vi "Main.vi"() -> ()   [LabVIEW 2017]
doc: "The myRIO Project template acquires acceleration data from the onboard accelerometer and displays the changes of acceleration values in a waveform chart."
uses:
  <vilib>/myRIO/Instrument Drivers/Onboard IO/DIO/typedefs/DIO Reference.ctl
  <vilib>/myRIO/Common/Instrument Driver Framework/Utilities/typedefs/myRIO Generic Hardware Reference.ctl
  <vilib>/myRIO/Common/Instrument Driver Framework/Utilities/typedefs/Hardware Version Enum.ctl
  <vilib>/myRIO/Common/Instrument Driver Framework/Utilities/typedefs/myRIO v1.0 Reference.ctl
  <vilib>/myRIO/Common/Instrument Driver Framework/Utilities/typedefs/Generic FPGA Reference.ctl
  <vilib>/myRIO/Common/Instrument Driver Framework/myRIO v1.0/DIO/typedefs/DIO Channels List.ctl
  <vilib>/myRIO/Common/Instrument Driver Framework/myRIO v1.0/DIO/typedefs/DIO Channels Enum.ctl
  <vilib>/userdefined/High Color/nirio_resource_hc.ctl
  <vilib>/myRIO/Instrument Drivers/Onboard IO/UART/typedef/VISA Configuration.ctl
  <vilib>/myRIO/Common/Instrument Driver Framework/Utilities/vis/Is FPGA Ref Available.vi
  <vilib>/myRIO/Common/Instrument Driver Framework/myRIO v1.0/DIO/vis/myRIO v1.1 Open DIO.vi
  <vilib>/myRIO/Instrument Drivers/Onboard IO/DIO/vis/Write.vi
  <vilib>/myRIO/Instrument Drivers/Onboard IO/DIO/vis/Read.vi
  <vilib>/myRIO/Common/Instrument Driver Framework/Utilities/vis/Validate Channels.vi
  <vilib>/myRIO/Common/Instrument Driver Framework/myRIO v1.0/DIO/vis/myRIO v1.0 Reserve DIO.vi
  <vilib>/myRIO/Common/Instrument Driver Framework/myRIO v1.0/UART/vis/myRIO v1.0 Close UART.vi
  <vilib>/myRIO/Common/Instrument Driver Framework/myRIO v1.0/Resource Manager/vis/myRIO v1.0 Reserve Channel List.vi
  <vilib>/myRIO/Common/Instrument Driver Framework/myRIO v1.0/DIO/vis/myRIO v1.0 Build MUX Configuration DIO.vi
  <vilib>/myRIO/Common/Instrument Driver Framework/myRIO v1.0/Resource Manager/vis/myRIO v1.0 Reserve Channel.vi
  <vilib>/myRIO/Common/Instrument Driver Framework/myRIO v1.0/Resource Manager/vis/myRIO v1.0 Unreserve Channel.vi
  <vilib>/myRIO/Common/Instrument Driver Framework/myRIO v1.0/Resource Manager/vis/myRIO v1.0 Create Configuration List.vi
  <vilib>/myRIO/Common/Instrument Driver Framework/myRIO v1.0/Resource Manager/vis/myRIO v1.0 Build Mutex Name.vi
  <vilib>/Utility/VariantDataType/GetNumericInfo.vi
  <vilib>/Utility/error.llb/Error Cluster From Error Code.vi
  <vilib>/myRIO/Common/Instrument Driver Framework/myRIO v1.0/myRIO v1.1 Open.vi
  <vilib>/myRIO/Common/Instrument Driver Framework/Utilities/vis/IO Manager.vi
  <vilib>/myRIO/Common/Instrument Driver Framework/Utilities/vis/Configuration Manager.vi
  <vilib>/myRIO/Common/Instrument Driver Framework/myRIO v1.0/Resource Manager/vis/myRIO v1.0 Configure IO.vi
  <vilib>/myRIO/Common/Instrument Driver Framework/myRIO v1.0/myRIO v1.0 Close.vi
  <vilib>/myRIO/Common/Instrument Driver Framework/myRIO v1.0/DIO/vis/myRIO v1.0 Write DIO.vi
  <vilib>/Instr/_visa.llb/VISA Configure Serial Port (Instr).vi
  <vilib>/myRIO/Common/Instrument Driver Framework/myRIO v1.0/DIO/vis/myRIO v1.0 Read DIO.vi
  <vilib>/Utility/file.llb/Write Delimited Spreadsheet (string).vi
  <vilib>/myRIO/Common/Instrument Driver Framework/Utilities/vis/FPGA Ref Manager.vi
  <vilib>/myRIO/Common/Instrument Driver Framework/myRIO v1.0/myRIO v1.0 Reset FPGA.vi
  <vilib>/myRIO/Common/Instrument Driver Framework/myRIO v1.0/IRQ/vis/myRIO v1.0 IRQ Info FGV.vi
  <vilib>/myRIO/Common/Instrument Driver Framework/myRIO v1.0/IRQ/vis/myRIO v1.0 Timer IRQ Info FGV.vi
  <vilib>/myRIO/Common/Instrument Driver Framework/myRIO v1.0/IRQ/vis/myRIO v1.0 ISR Agent.vi
  <vilib>/myRIO/Express VI/Onboard IO/DO/DO Express VI.xnode
  <vilib>/myRIO/Instrument Drivers/Onboard IO/DIO/vis/myRIO DIO Open.xnode
  <vilib>/myRIO/Express VI/Onboard Devices/LED/LED Express VI.xnode
  <vilib>/myRIO/Express VI/Onboard IO/UART/UART Express VI.xnode
  <vilib>/myRIO/Express VI/Onboard IO/DI/DI Express VI.xnode
  <vilib>/myRIO/Express VI/Onboard Devices/Button/Button Express VI.xnode
  <vilib>/myRIO/Instrument Drivers/Utilities/Utilities.lvlib
  <vilib>/myRIO/Instrument Drivers/Onboard IO/UART/UART.lvlib
  <vilib>/myRIO/Instrument Drivers/Onboard IO/DIO/DIO.lvlib
panel:
  out "LinkIt Response\nTimed Out 3":bool
  out "time to \nrespond":dbl
  out "DIO Failure":bool
  out "System Log":string
  out "Data Log":string[](array[string])
  out "System Log Write Path":path
  out "Data Log Write Path":path
  out "Pin 11 State":bool
  out "Pin 13 State":bool
  out "Message Received":string
  out "Message to Send":string
  out "Time to Send \nMessage":dbl
  out "LinkIt Response\nTimed Out 2":bool
  out "LinkIt Response\nTimed Out 1":bool
  out "Data Queue Error":bool
  out "LinkIt Failure":bool
  out "Initialisation \nsuccessfull":bool
  out "Storage Device Failure":bool
  out "D.L.B. Status":bool
  out "?":i32(slide) scale=0.1..100.0
  out "?":bool
  out "?":bool
  out "?":bool
  out "?":bool
  out "S.L.H. Status":bool
  out "S.L.B. Status":bool
  out "S.L. Status":bool
  out "D.L.H. Status":bool
  out "M.S. Status":bool
  out "M.H. Status":bool
  out "M.R. Status":bool
  out "System Uptime":string
  in  "Array":string[](array[string])
  out "error out":errorcluster
  in  "Stop":bool
  # "Overview: The myRIO Project template acquires acceleration data from the onboard accelerometer and displays the changes of acceleration values in a waveform chart.\nInstructions:\n1. Check the myRIO target IP address in the project and make sure the target IP address is correct. \n2. Run this VI."
  # "Signal Level"
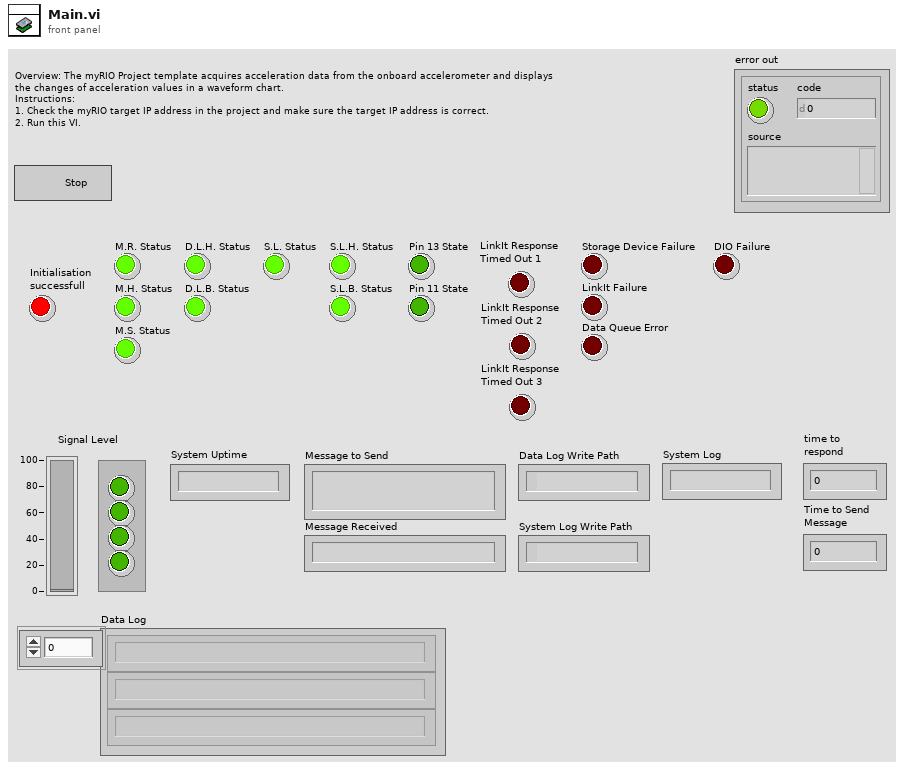
[diagram p1: front panel]
types:
  T1 = cluster{string, string, string, string, string, string, string, string, string, string}
  T2 = typedef "DIO.lvlib/DIO Reference.ctl" = cluster{"myRIO Reference":T3, "DIO Channels List":T7}
  T3 = typedef "myRIO Generic Hardware Reference.ctl" = cluster{"myRIO Model":T4, "myRIO Hardware Reference":T5}
  T4 = typedef "Hardware Version Enum.ctl" = enum16{"Unknown", "myRIO-1900", "myRIO-1950", "roboRIO", "NI ELVIS RIO CM"}
  T5 = typedef "myRIO v1.0 Reference.ctl" = cluster{"Generic FPGA Reference":T6, "Allow multiple opens":bool}
  T6 = typedef "Generic FPGA Reference.ctl" = refnum<k20>
  T7 = typedef "DIO Channels List.ctl" = T8[]
  T8 = typedef "DIO Channels Enum.ctl" = enum16{"Not Connected", "C/DIO0", "C/DIO1", "C/DIO2", "C/DIO3", "C/DIO4", "C/DIO5", "C/DIO6", "C/DIO7", "A/DIO0", "A/DIO1", "A/DIO2", "A/DIO3", "A/DIO4", "A/DIO5", "A/DIO6", "A/DIO7", "A/DIO8", "A/DIO9", "A/DIO10", "A/DIO11", "A/DIO12", "A/DIO13", "A/DIO14", "A/DIO15", "B/DIO0", "B/DIO1", "B/DIO2", "B/DIO3", "B/DIO4", "B/DIO5", "B/DIO6", "B/DIO7", "B/DIO8", "B/DIO9", "B/DIO10", "B/DIO11", "B/DIO12", "B/DIO13", "B/DIO14", "B/DIO15", "LED0", "LED1", "LED2", "LED3", "Button0", "DIO/DIO0", "DIO/DIO1", "DIO/DIO2", "DIO/DIO3", "DIO/DIO4", "DIO/DIO5", "DIO/DIO6", "DIO/DIO7", "DIO/DIO8", "DIO/DIO9", "SPI/CS0", "SPI/CS1", "SPI/CS2", "SPI/CS3", "LED RADIO (Green)", "LED RADIO (Red)", "LED COMM (Green)", "LED COMM (Red)", "LED MODE (Green)", "LED MODE (Red)"}
  T9 = typedef "nirio_resource_hc.ctl" = tag
  T10 = typedef "UART.lvlib/VISA Configuration.ctl" = cluster{"baud rate (9600)":u32, "data bits (8)":u16, "parity (0:none)":enum16{"None", "Odd", "Even", "Mark", "Space"}, "stop bits (10: 1 bit)":u16, "flow control (0:none)":u16, "termination char\n(0xA = '\\n' = LF) ":u8, "Enable Termination\nChar (T)":bool, "timeout (10sec)":u32}
  T11 = enum16{"open", "replace", "create", "open or create", "replace or create", "replace or create with confirmation"}
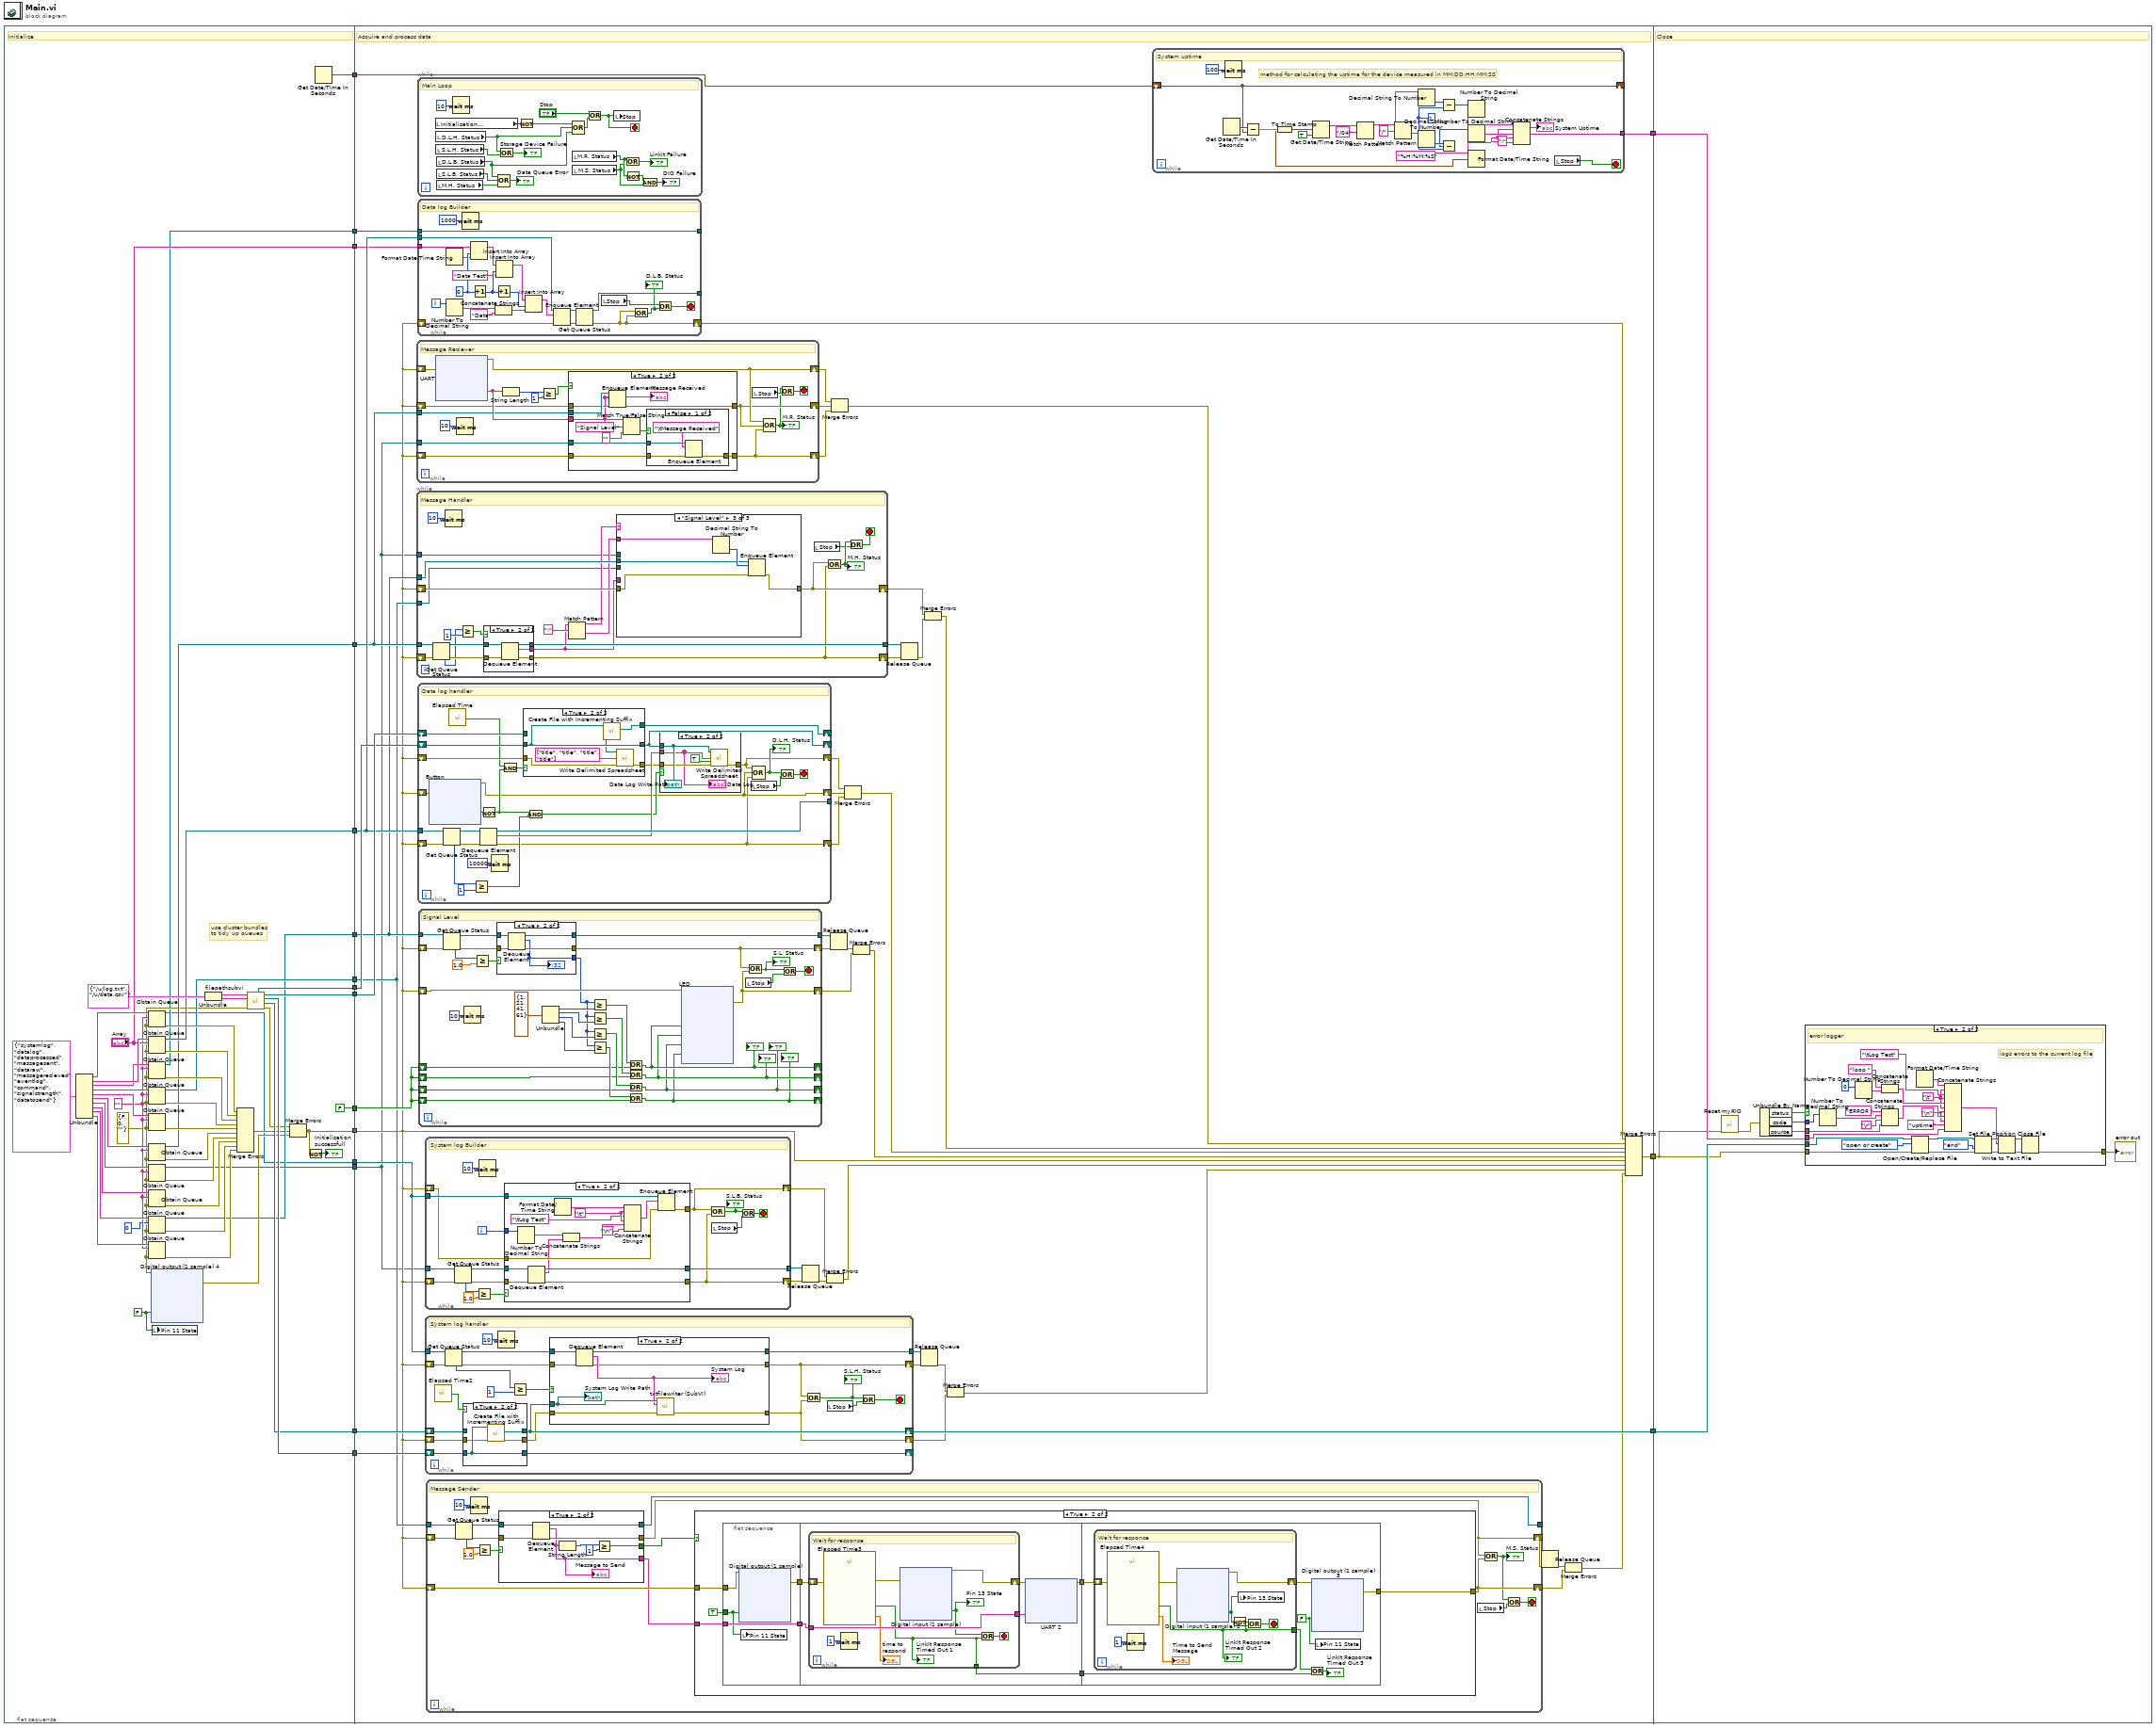
[diagram p0: block diagram]
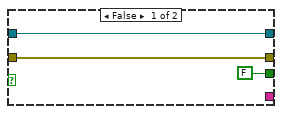
[diagram p3: hidden frame]
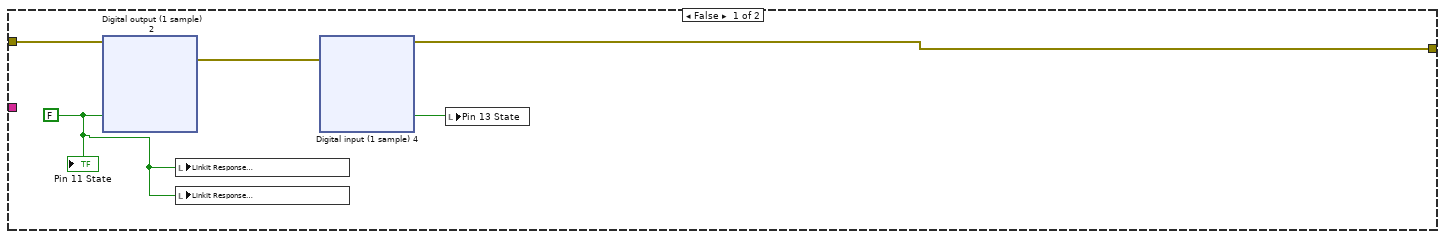
[diagram p4: hidden frame]
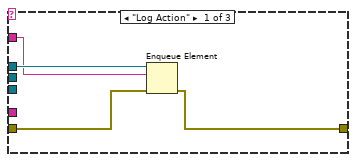
[diagram p6: hidden frame]
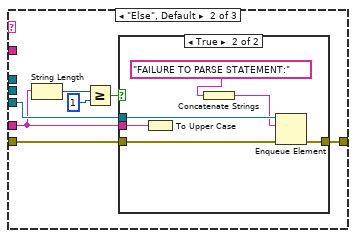
[diagram p7: hidden frame]
diagram:
  n1 = flat-sequence {
    tunnel: [w64] -> w17
    tunnel: [w55] -> w16
    tunnel: [w21] -> w15
    tunnel: [w54] -> w14
    tunnel: [w53] -> w13
    tunnel: [w19] -> w12
    tunnel: ["Array"] -> w11
    tunnel: [w20] -> w10
    tunnel: [w37] -> w9
    tunnel: [w36] -> w8
    tunnel: [w34] -> w6
    tunnel: [w33] -> w5
    tunnel: [w31] -> w4
    tunnel: [w30] -> w3
    tunnel: [FALSE] -> w2
    tunnel: [w152] -> w18
    tunnel: w17 -> [w151]
    tunnel: w16 -> [w148]
    tunnel: w15 -> [w111]
    tunnel: w14 -> [w150]
    tunnel: w13 -> [w149]
    tunnel: w12 -> [w141]
    tunnel: w11 -> [w147]
    tunnel: w10 -> [w146]
    tunnel: w9 -> [w145]
    tunnel: w8 -> [w144]
    tunnel: [w143] -> w7
    tunnel: w6 -> [w142]
    tunnel: w5 -> [w113]
    tunnel: w4 -> [w102]
    tunnel: w3 -> [w116]
    tunnel: w2 -> [w138]
    tunnel: [w101] -> w1
    tunnel: w18 -> [w857]
    tunnel: w7 -> [w854]
    tunnel: w1 -> [w853]
    frame #0 {
      w24 = FALSE
      w32 = ""
      w23 = errorcluster {"status"=FALSE, "code"=0, "source"=""} ("error in (no error)")
      # "use cluster bundles\nto tidy up queues"
      # "Initialize"
      n2 = Unbundle(T1 {"systemlog", "datalog", "dataprocessed", "messagesent", "dataraw", "messagerecieved", "eventlog", "command", "signalstrength", "datatosend"}) -> (w60:string, w59:string, w58:string, w57:string, w56:string, w47:string, w45:string, w44:string, w43:string, w42:string)
      n3 = Obtain Queue(name (unnamed)=w60, element data type=w32, error in (no error)=w23) -> (queue out=w19:refnum<queue>, error out=w52:errorcluster)  [unwired: 2 in, 1 out]
      n4 = Obtain Queue(name (unnamed)=w59, element data type="Array", error in (no error)=w23) -> (queue out=w55:refnum<queue>, error out=w51:errorcluster)  [unwired: 2 in, 1 out]
      n5 = Obtain Queue(name (unnamed)=w58, element data type=w32, error in (no error)=w23) -> (queue out=w20:refnum<queue>, error out=w50:errorcluster)  [unwired: 2 in, 1 out]
      n6 = Obtain Queue(name (unnamed)=w57, element data type=w32, error in (no error)=w23) -> (queue out=w33:refnum<queue>, error out=w49:errorcluster)  [unwired: 2 in, 1 out]
      n7 = Obtain Queue(name (unnamed)=w56, element data type=w32, error in (no error)=w23) -> (error out=w48:errorcluster)  [unwired: 2 in, 2 out]
      n8 = Obtain Queue(name (unnamed)=w47, element data type=w32, error in (no error)=w23) -> (queue out=w34:refnum<queue>, error out=w46:errorcluster)  [unwired: 2 in, 1 out]
      n9 = Obtain Queue(name (unnamed)=w45, element data type=w32, error in (no error)=w23) -> (queue out=w31:refnum<queue>, error out=w41:errorcluster)  [unwired: 2 in, 1 out]
      n10 = Obtain Queue(name (unnamed)=w44, element data type=w32, error in (no error)=w23) -> (error out=w40:errorcluster)  [unwired: 2 in, 2 out]
      n11 = Obtain Queue(name (unnamed)=w43, element data type=0, error in (no error)=w23) -> (queue out=w30:refnum<queue>, error out=w39:errorcluster)  [unwired: 2 in, 1 out]
      n12 = Obtain Queue(name (unnamed)=w42, element data type=w32, error in (no error)=w23) -> (error out=w38:errorcluster)  [unwired: 2 in, 2 out]
      n13 = xnode ("Digital output (1 sample) 4")("A/DIO0 (Pin 11)"=w24, "error in (no error)"=w23) -> ("error out"=w22:errorcluster)
      n14 = local write "Pin 11 State"(w24) -> ()
      n15 = Unbundle(cluster{string, string} {"/u/log.txt", "/u/data.csv"}) -> (w62:string, w61:string)
      n16 = Merge Errors(w52, w51, w50, w49, w48, w46, w41, w40, w39, w38) -> (w26:errorcluster)
      n17 = call "filepathsubvi.vi"("error in (no error)"=w23, "String"=w61, "String 2"=w62) -> ("error out"=w25:errorcluster, "actual path"=w36:path, "Path"=w37:path, "actual path 2"=w54:path, "Path 2"=w53:path)  [unwired: 4 in]
      n18 = Merge Errors(w25, w26, w22) -> (w21:errorcluster)
      n19 = Not(x=w21) -> (.not. x?=→"Initialisation \nsuccessfull":bool)
      n20 = Get Date/Time In Seconds() -> (seconds since 1Jan1904=w64:timestamp)
    }
    frame #1 {
      # "Acquire and process data"
      n21 = while {
        shift-right: [w588] -> w123
        shift-left: w111 -> [w600]
        tunnel: w142 -> [w592]
        shift-right: [w587] -> w122
        shift-left: w111 -> [w591]
        shift-right: [w586] -> w121
        shift-left: w111 -> [w590]
        tunnel: w102 -> [w589]
        stop <- w597 stop-if-true
        # "Message Reciever"
        n22 = xnode "UART"("error in (no error)"=w600) -> ("Characters Read"=w593:string, "error out"=w588:errorcluster)
        n23 = Wait (ms)(milliseconds to wait=u32 10) -> ()  [unwired: 1 out]
        n24 = String Length(string=w593) -> (length=w595:i32)
        n25 = Greater Or Equal?(x=w595, y=1) -> (x >= y?=w596:bool)
        n26 = case shown="True" w596 {
          tunnel: w593 -> [_ w606]
          tunnel: w592 -> [_ w612]
          tunnel: w591 -> [w602 w611]
          tunnel: [w602 w610] -> w587
          tunnel: [w601 w609] -> w586
          tunnel: w590 -> [w601 w608]
          tunnel: w589 -> [_ w607]
          frame False {
          }
          frame True {
            n27 = Enqueue Element(queue=w612, element=w606, error in (no error)=w611) -> (error out=w610:errorcluster)  [unwired: 1 in, 2 out]
            n28 = Match True/False String(2:"" ("false string"), 3:"Signal Level" ("true string"), 4:w606) -> (0:w604:bool)  [unwired: 1 out]
            n29 = case shown="False" w604 {
              tunnel: [w615 w617] -> w609
              tunnel: w608 -> [w614 w617]
              tunnel: w607 -> [w613 _]
              frame False {
                n30 = Enqueue Element(queue=w613, element="\tMessage Received", error in (no error)=w614) -> (error out=w615:errorcluster)  [unwired: 1 in, 2 out]
              }
              frame True {
              }
            }
            "Message Received" <- w606
          }
        }
        n31 = local read "Stop"() -> (w598:bool)
        n32 = Compound Arithmetic op=OR(w588, w587, w586) -> (w585:bool)
        "M.R. Status" <- w585
        n33 = Or(x=w585, y=w598) -> (x .or. y?=w597:bool)
      }
      n34 = while {
        tunnel: [w553] -> w117
        tunnel: w142 -> [w552]
        shift-right: [w541] -> w118
        shift-left: w111 -> [w539]
        shift-right: [w546] -> w119
        shift-left: w111 -> [w550]
        tunnel: w116 -> [w549]
        tunnel: w113 -> [w542]
        tunnel: w102 -> [w533]
        stop <- w545 stop-if-true
        # "Message Handler"
        n35 = Get Queue Status(queue=w552, error in (no error)=w539) -> (queue out=w540:refnum<queue>, error out=w538:errorcluster, # elements in queue=w535:i32)  [unwired: 1 in, 5 out]
        n36 = Wait (ms)(milliseconds to wait=u32 10) -> ()  [unwired: 1 out]
        n37 = Greater Or Equal?(x=w535, y=1) -> (x >= y?=w536:bool)
        n38 = case shown="True" w536 {
          tunnel: [w556 w561] -> w553
          tunnel: [_ w560] -> w534
          tunnel: [w555 w559] -> w541
          tunnel: w540 -> [w556 w558]
          tunnel: w538 -> [w555 w557]
          frame False {
          }
          frame True {
            n39 = Dequeue Element(queue=w558, error in (no error)=w557) -> (queue out=w561:refnum<queue>, element=w560:string, error out=w559:errorcluster)  [unwired: 1 in, 1 out]
          }
        }
        n40 = Match Pattern(string=w534, regular expression=":") -> (before substring=w547:string, after substring=w548:string)  [unwired: 1 in, 2 out]
        n41 = case shown="\"Signal Level\"" w547 {
          tunnel: w548 -> [w562 _ w583]
          tunnel: w550 -> [w565 w571 w582]
          tunnel: [w563 w570 w581] -> w546
          tunnel: w549 -> [_ _ w580]
          tunnel: w534 -> [_ w567 _]
          tunnel: w542 -> [_ w572 _]
          tunnel: w533 -> [w564 _ _]
          frame "Log Action" {
            n42 = Enqueue Element(queue=w564, element=w562, error in (no error)=w565) -> (error out=w563:errorcluster)  [unwired: 1 in, 2 out]
          }
          frame "Else", Default {
            n43 = String Length(string=w567) -> (length=w568:i32)
            n44 = Greater Or Equal?(x=w568, y=1) -> (x >= y?=w566:bool)
            n45 = case shown="True" w566 {
              tunnel: w572 -> [_ w579]
              tunnel: w571 -> [w573 w578]
              tunnel: [w573 w577] -> w570
              tunnel: w567 -> [_ w575]
              frame False {
              }
              frame True {
                n46 = To Upper Case(1:w575) -> ()  [unwired: 1 out]
                n47 = Concatenate Strings("FAILURE TO PARSE STATEMENT:") -> (w576:string)
                n48 = Enqueue Element(queue=w579, element=w576, error in (no error)=w578) -> (error out=w577:errorcluster)  [unwired: 1 in, 2 out]
              }
            }
          }
          frame "Signal Level" {
            n49 = Decimal String To Number(string=w583) -> (number=w584:i32)  [unwired: 2 in, 1 out]
            n50 = Enqueue Element(queue=w580, element=w584, error in (no error)=w582) -> (error out=w581:errorcluster)  [unwired: 1 in, 2 out]
          }
        }
        n51 = local read "Stop"() -> (w543:bool)
        n52 = Compound Arithmetic op=OR(w546, w541) -> (w544:bool)
        "M.H. Status" <- w544
        n53 = Or(x=w544, y=w543) -> (x .or. y?=w545:bool)
      }
      n54 = while {
        stop <- w844 stop-if-true
        # "Main Loop"
        n55 = local read "Initialisation \nsuccessfull"() -> (w847:bool)
        n56 = local read "D.L.H. Status"() -> (w850:bool)
        n57 = local read "S.L.H. Status"() -> (w849:bool)
        n58 = local read "D.L.B. Status"() -> (w841:bool)
        n59 = local read "S.L.B. Status"() -> (w840:bool)
        n60 = local read "M.H. Status"() -> (w846:bool)
        n61 = Wait (ms)(milliseconds to wait=u32 10) -> ()  [unwired: 1 out]
        n62 = Compound Arithmetic op=OR(w841, w840, w846) -> (→"Data Queue Error":bool)
        n63 = Or(x=w850, y=w849) -> (x .or. y?=→"Storage Device Failure":bool)
        n64 = Not(x=w847) -> (.not. x?=w842:bool)
        n65 = Compound Arithmetic op=OR(w842, w850, w841) -> (w843:bool)
        n66 = local read "M.R. Status"() -> (w837:bool)
        n67 = local read "M.S. Status"() -> (w836:bool)
        n68 = Or(x="Stop", y=w843) -> (x .or. y?=w844:bool)
        n69 = local write "Stop"(w844) -> ()
        n70 = Or(x=w837, y=w836) -> (x .or. y?=→"LinkIt Failure":bool)
        n71 = Not(x=w837) -> (.not. x?=w838:bool)
        n72 = And(x=w838, y=w836) -> (x .and. y?=→"DIO Failure":bool)
      }
      n73 = while {
        tunnel: w148 -> [w696]
        tunnel: [w693] -> _
        tunnel: [w677] -> _
        tunnel: w146 -> [w677]
        tunnel: w147 -> [w676]
        shift-right: [w675] -> w110
        shift-left: w111 -> [w692]
        i -> [w680]
        stop <- w679 stop-if-true
        w688 = 0
        # "Data log Builder"
        n74 = Format Date/Time String() -> (date/time string=w685:string)  [unwired: 3 in]
        n75 = Number To Decimal String(number=w680) -> (decimal integer string=w683:string)  [unwired: 1 in]
        n76 = Wait (ms)(milliseconds to wait=u32 1000) -> ()  [unwired: 1 out]
        n77 = Insert Into Array(array=w676, index=w688, new element=w685) -> (w691:string[])
        n78 = Increment(x=w688) -> (x+1=w687:i32)
        n79 = Concatenate Strings(w683, "Data") -> (w681:string)
        n80 = Insert Into Array(array=w691, index=w687, new element="Data Test" ("text")) -> (w690:string[])
        n81 = Increment(x=w687) -> (x+1=w686:i32)
        n82 = Insert Into Array(array=w690, index=w686, new element=w681) -> (w689:string[])
        n83 = Enqueue Element(queue=w696, element=w689, error in (no error)=w692) -> (queue out=w694:refnum<queue>, error out=w695:errorcluster)  [unwired: 1 in, 1 out]
        n84 = Get Queue Status(queue=w694, error in (no error)=w695) -> (queue out=w693:refnum<queue>, error out=w675:errorcluster)  [unwired: 1 in, 6 out]
        n85 = local read "Stop"() -> (w678:bool)
        n86 = Compound Arithmetic op=OR(w675, w675) -> (w674:bool)
        "D.L.B. Status" <- w674
        n87 = Or(x=w678, y=w674) -> (x .or. y?=w679:bool)
      }
      n88 = while {
        shift-right: [w752] -> w114
        shift-left: w111 -> [w748]
        tunnel: w148 -> [w760]
        tunnel: [w758] -> _
        shift-right: [w747] -> _
        shift-left: w149 -> [w746]
        shift-right: [w743] -> _
        shift-left: w150 -> [w744]
        shift-right: [w734] -> w120
        shift-left: w111 -> [w759]
        shift-right: [w735] -> w115
        shift-left: w111 -> [w736]
        stop <- w749 stop-if-true
        # "Data log handler"
        n89 = xnode "Button"("error in (no error)"=w736) -> ("Value"=w742:bool, "error out"=w735:errorcluster)
        n90 = Get Queue Status(queue=w760, error in (no error)=w759) -> (queue out=w757:refnum<queue>, error out=w756:errorcluster, # elements in queue=w755:i32)  [unwired: 1 in, 5 out]
        n91 = call "Elapsed Time"() -> ("Time has Elapsed"=w741:bool)  [unwired: 12 in, 7 out]
        n92 = Greater Or Equal?(x=w755, y=1) -> (x >= y?=w738:bool)
        n93 = Dequeue Element(queue=w757, error in (no error)=w756) -> (queue out=w758:refnum<queue>, element=w750:string[], error out=w734:errorcluster)  [unwired: 1 in, 1 out]
        n94 = Not(x=w742) -> (.not. x?=w739:bool)
        n95 = Wait (ms)(milliseconds to wait=u32 10000) -> ()  [unwired: 1 out]
        n96 = And(x=w741, y=w739) -> (x .and. y?=w740:bool)
        n97 = case shown="True" w740 {
          tunnel: w748 -> [w798 w804]
          tunnel: [w799 w801] -> w747
          tunnel: w746 -> [w799 w801]
          tunnel: [w798 w803] -> w745
          tunnel: w744 -> [w797 _]
          tunnel: [w797 w800] -> w743
          frame False {
          }
          frame True {
            n98 = call <vilib>:"Create File with Incrementing Suffix.vi"("file path"=w801) -> ("actual path"=w800:path)  [unwired: 8 in, 2 out]
            n99 = call-poly <vilib>:"Write Delimited Spreadsheet.vi"("file path (dialog if empty)"=w800, "1D data"=string[] ["title", "title", "title", "title"], "error in (no error)"=w804) -> ("error out"=w803:errorcluster)  [unwired: 11 in, 1 out]
          }
        }
        n100 = And(x=w739, y=w738) -> (x .and. y?=w737:bool)
        n101 = case shown="True" w737 {
          tunnel: w745 -> [w805 w809]
          tunnel: w747 -> [_ w810]
          tunnel: [w805 w808] -> w752
          tunnel: w750 -> [_ w806]
          frame False {
          }
          frame True {
            n102 = call-poly <vilib>:"Write Delimited Spreadsheet.vi"("file path (dialog if empty)"=w810, "1D data"=w806, "append to file? (new file:F)"=TRUE, "error in (no error)"=w809) -> ("error out"=w808:errorcluster)  [unwired: 10 in, 1 out]
            "Data Log Write Path" <- w810
            "Data Log" <- w806
          }
        }
        n103 = local read "Stop"() -> (w751:bool)
        n104 = Compound Arithmetic op=OR(w752, w735, w734) -> (w753:bool)
        "D.L.H. Status" <- w753
        n105 = Or(x=w753, y=w751) -> (x .or. y?=w749:bool)
      }
      n106 = while {
        shift-right: [w158] -> w135
        shift-left: w111 -> [w169]
        shift-right: [w157] -> w126
        shift-left: w111 -> [w185]
        shift-right: [w162] -> _
        shift-left: w138 -> [w180]
        shift-right: [w161] -> _
        shift-left: w138 -> [w179]
        shift-right: [w160] -> _
        shift-left: w138 -> [w178]
        shift-right: [w159] -> _
        shift-left: w138 -> [w177]
        tunnel: w116 -> [w170]
        tunnel: [w168] -> w134
        stop <- w155 stop-if-true
        # "Signal Level"
        n107 = Get Queue Status(queue=w170, error in (no error)=w169) -> (queue out=w174:refnum<queue>, error out=w175:errorcluster, # elements in queue=w172:i32)  [unwired: 1 in, 5 out]
        n108 = Wait (ms)(milliseconds to wait=u32 10) -> ()  [unwired: 1 out]
        n109 = Greater Or Equal?(x=w172, y=1.0) -> (x >= y?=w173:bool)
        n110 = case shown="True" w173 {
          tunnel: w174 -> [w187 w192]
          tunnel: w175 -> [w186 w191]
          tunnel: [w187 w190] -> w168
          tunnel: [_ w188] -> w153
          tunnel: [w186 w189] -> w158
          frame False {
          }
          frame True {
            n111 = Dequeue Element(queue=w192, error in (no error)=w191) -> (queue out=w190:refnum<queue>, element=w188:i32, error out=w189:errorcluster)  [unwired: 1 in, 1 out]
            "?" <- w188
          }
        }
        n112 = Unbundle(cluster{i32, i32, i32, i32} {1, 21, 41, 61}) -> (w166:i32, w165:i32, w164:i32, w163:i32)
        n113 = Greater Or Equal?(x=w153, y=w166) -> (x >= y?=w184:bool)
        n114 = Greater Or Equal?(x=w153, y=w165) -> (x >= y?=w183:bool)
        n115 = Greater Or Equal?(x=w153, y=w164) -> (x >= y?=w182:bool)
        n116 = Greater Or Equal?(x=w153, y=w163) -> (x >= y?=w181:bool)
        n117 = Or(x=w184, y=w180) -> (x .or. y?=w162:bool)
        "?" <- w162
        n118 = Or(x=w183, y=w179) -> (x .or. y?=w161:bool)
        "?" <- w161
        n119 = Or(x=w182, y=w178) -> (x .or. y?=w160:bool)
        "?" <- w160
        n120 = Or(x=w181, y=w177) -> (x .or. y?=w159:bool)
        "?" <- w159
        n121 = xnode "LED"("61+"=w162, "41-60"=w161, "21-40"=w160, "1-20"=w159, "error in (no error)"=w185) -> ("error out"=w157:errorcluster)
        n122 = local read "Stop"() -> (w156:bool)
        n123 = Compound Arithmetic op=OR(w158, w157) -> (w154:bool)
        "S.L. Status" <- w154
        n124 = Or(x=w154, y=w156) -> (x .or. y?=w155:bool)
      }
      n125 = while {
        shift-right: [w701] -> w130
        shift-left: w111 -> [w702]
        tunnel: w102 -> [w707]
        tunnel: [w705] -> w140
        shift-right: [w700] -> w139
        shift-left: w111 -> [w706]
        tunnel: w141 -> [w703]
        i -> [w698]
        stop <- w712 stop-if-true
        # "System log Builder"
        n126 = Get Queue Status(queue=w707, error in (no error)=w706) -> (queue out=w709:refnum<queue>, error out=w708:errorcluster, # elements in queue=w711:i32)  [unwired: 1 in, 5 out]
        n127 = Greater Or Equal?(x=w711, y=1.0) -> (x >= y?=w704:bool)
        n128 = Wait (ms)(milliseconds to wait=u32 10) -> ()  [unwired: 1 out]
        n129 = case shown="True" w704 {
          tunnel: w709 -> [w716 w733]
          tunnel: w708 -> [w717 w732]
          tunnel: [w716 w731] -> w705
          tunnel: [w717 w730] -> w700
          tunnel: w698 -> [_ w723]
          tunnel: w703 -> [_ w722]
          tunnel: w702 -> [w715 w720]
          tunnel: [w715 w718] -> w701
          frame False {
          }
          frame True {
            w726 = "\t"
            n130 = Number To Decimal String(number=w723) -> (decimal integer string=w727:string)  [unwired: 1 in]
            n131 = Dequeue Element(queue=w733, error in (no error)=w732) -> (queue out=w731:refnum<queue>, element=w719:string, error out=w730:errorcluster)  [unwired: 1 in, 1 out]
            n132 = Format Date/Time String() -> (date/time string=w728:string)  [unwired: 3 in]
            n133 = Concatenate Strings(w727, w719) -> (w729:string)
            n134 = Concatenate Strings(w728, w726, "\tLog Test" ("text"), w726, w729, "\n") -> (w721:string)
            n135 = Enqueue Element(queue=w722, element=w721, error in (no error)=w720) -> (error out=w718:errorcluster)  [unwired: 1 in, 2 out]
          }
        }
        n136 = Compound Arithmetic op=OR(w701, w700) -> (w699:bool)
        "S.L.B. Status" <- w699
        n137 = local read "Stop"() -> (w713:bool)
        n138 = Or(x=w699, y=w713) -> (x .or. y?=w712:bool)
      }
      n139 = while {
        shift-right: [w637] -> w129
        shift-left: w111 -> [w641]
        tunnel: w141 -> [w654]
        shift-right: [w643] -> w143
        shift-left: w144 -> [w645]
        shift-right: [w642] -> _
        shift-left: w145 -> [w644]
        shift-right: [w636] -> w132
        shift-left: w111 -> [w653]
        tunnel: [w635] -> w133
        stop <- w647 stop-if-true
        # "System log handler"
        n140 = call "Elapsed Time2"() -> ("Time has Elapsed"=w646:bool)  [unwired: 12 in, 7 out]
        n141 = Get Queue Status(queue=w654, error in (no error)=w653) -> (queue out=w639:refnum<queue>, error out=w638:errorcluster, # elements in queue=w652:i32)  [unwired: 1 in, 5 out]
        n142 = case shown="True" w646 {
          tunnel: w644 -> [w658 w661]
          tunnel: [w657 w662] -> w643
          tunnel: [w658 w661] -> w642
          tunnel: w645 -> [w657 _]
          tunnel: w641 -> [w656 w660]
          tunnel: [w656 w659] -> w640
          frame False {
          }
          frame True {
            n143 = call <vilib>:"Create File with Incrementing Suffix.vi"("error in (no error)"=w660, "file path"=w661) -> ("error out"=w659:errorcluster, "actual path"=w662:path)  [unwired: 7 in, 1 out]
          }
        }
        n144 = Wait (ms)(milliseconds to wait=u32 10) -> ()  [unwired: 1 out]
        n145 = Greater Or Equal?(x=w652, y=1) -> (x >= y?=w650:bool)
        n146 = case shown="True" w650 {
          tunnel: w640 -> [w665 w673]
          tunnel: w643 -> [_ w672]
          tunnel: [w665 w671] -> w637
          tunnel: w639 -> [w663 w670]
          tunnel: w638 -> [w664 w669]
          tunnel: [w664 w667] -> w636
          tunnel: [w663 w666] -> w635
          frame False {
          }
          frame True {
            n147 = Dequeue Element(queue=w670, error in (no error)=w669) -> (queue out=w666:refnum<queue>, element=w668:string, error out=w667:errorcluster)  [unwired: 1 in, 1 out]
            "System Log" <- w668
            n148 = call "txtfilewriter (SubVI).vi"("error in (no error)"=w673, "String"=w668, "actual path"=w672) -> ("error out"=w671:errorcluster)  [unwired: 8 in]
            "System Log Write Path" <- w672
          }
        }
        n149 = Compound Arithmetic op=OR(w636, w637) -> (w649:bool)
        "S.L.H. Status" <- w649
        n150 = local read "Stop"() -> (w648:bool)
        n151 = Or(x=w649, y=w648) -> (x .or. y?=w647:bool)
      }
      n152 = while {
        shift-right: [w235] -> w124
        shift-left: w111 -> [w247]
        tunnel: w113 -> [w238]
        tunnel: [w242] -> w137
        shift-right: [w234] -> w136
        shift-left: w111 -> [w237]
        stop <- w231 stop-if-true
        # "Message Sender"
        n153 = Get Queue Status(queue=w238, error in (no error)=w237) -> (queue out=w239:refnum<queue>, error out=w236:errorcluster, # elements in queue=w244:i32)  [unwired: 1 in, 5 out]
        n154 = Wait (ms)(milliseconds to wait=u32 10) -> ()  [unwired: 1 out]
        n155 = Greater Or Equal?(x=w244, y=1.0) -> (x >= y?=w240:bool)
        n156 = case shown="True" w240 {
          tunnel: w239 -> [w250 w256]
          tunnel: w236 -> [w249 w255]
          tunnel: [FALSE w254] -> w243
          tunnel: [w250 w253] -> w242
          tunnel: [_ w251] -> w241
          tunnel: [w249 w252] -> w234
          frame False {
          }
          frame True {
            n157 = Dequeue Element(queue=w256, error in (no error)=w255) -> (queue out=w253:refnum<queue>, element=w251:string, error out=w252:errorcluster)  [unwired: 1 in, 1 out]
            "Message to Send" <- w251
            n158 = String Length(string=w251) -> (length=w258:i32)
            n159 = Greater Or Equal?(x=w258, y=1) -> (x >= y?=w254:bool)
          }
        }
        n160 = case shown="True" w243 {
          tunnel: w241 -> [_ w340]
          tunnel: w247 -> [w263 w338]
          tunnel: [w261 w335] -> w235
          frame False {
            w259 = FALSE
            n161 = xnode "Digital output (1 sample) 2"("A/DIO0 (Pin 11)"=w259, "error in (no error)"=w263) -> ("error out"=w262:errorcluster)
            n162 = local write "LinkIt Response\nTimed Out 1"(w259) -> ()
            n163 = local write "LinkIt Response\nTimed Out 2"(w259) -> ()
            n164 = xnode "Digital input (1 sample) 4"("error in (no error)"=w262) -> ("A/DIO1 (Pin 13)"=w260:bool, "error out"=w261:errorcluster)
            n165 = local write "Pin 13 State"(w260) -> ()
            "Pin 11 State" <- w259
          }
          frame True {
            n166 = flat-sequence {
              tunnel: w340 -> [w345]
              tunnel: [w345] -> w341
              tunnel: TRUE -> [w342]
              tunnel: w338 -> [w344]
              tunnel: [w343] -> w337
              tunnel: w341 -> [w385]
              tunnel: w337 -> [w384]
              tunnel: [w382] -> w336
              tunnel: [w381] -> w334
              tunnel: w336 -> [w453]
              tunnel: [w451] -> w335
              tunnel: w334 -> [w447]
              frame #0 {
                n167 = xnode "Digital output (1 sample)"("A/DIO0 (Pin 11)"=w342, "error in (no error)"=w344) -> ("error out"=w343:errorcluster)
                n168 = local write "Pin 11 State"(w342) -> ()
              }
              frame #1 {
                n169 = while {
                  tunnel: w385 -> [w395]
                  tunnel: [w395] -> w386
                  shift-right: [w393] -> w383
                  shift-left: w384 -> [w392]
                  tunnel: [w387] -> w381
                  stop <- w389 stop-if-true
                  # "Wait for response"
                  n170 = call "Elapsed Time3"("error in (no error)"=w392) -> ("Elapsed Time (s)"=→"time to \nrespond":dbl, "Time has Elapsed"=w387:bool, "error out"=w391:errorcluster)  [unwired: 11 in, 5 out]
                  "LinkIt Response\nTimed Out 1" <- w387
                  n171 = Wait (ms)(milliseconds to wait=u32 1) -> ()  [unwired: 1 out]
                  n172 = xnode "Digital input (1 sample)"("error in (no error)"=w391) -> ("A/DIO1 (Pin 13)"=w390:bool, "error out"=w393:errorcluster)
                  "Pin 13 State" <- w390
                  n173 = Or(x=w390, y=w387) -> (x .or. y?=w389:bool)
                }
                n174 = xnode "UART 2"("Characters to Write"=w386, "error in (no error)"=w383) -> ("error out"=w382:errorcluster)  [unwired: 1 out]
              }
              frame #2 {
                w450 = FALSE ("A/DIO0 (Pin 11)")
                n175 = while {
                  shift-right: [w495] -> w452
                  shift-left: w453 -> [w496]
                  tunnel: [w489] -> w448
                  stop <- w493 stop-if-true
                  # "Wait for responce"
                  n176 = call "Elapsed Time4"("error in (no error)"=w496) -> ("Elapsed Time (s)"=→"Time to Send \nMessage":dbl, "Time has Elapsed"=w489:bool, "error out"=w492:errorcluster)  [unwired: 11 in, 5 out]
                  "LinkIt Response\nTimed Out 2" <- w489
                  n177 = Wait (ms)(milliseconds to wait=u32 1) -> ()  [unwired: 1 out]
                  n178 = xnode "Digital input (1 sample) 2"("error in (no error)"=w492) -> ("A/DIO1 (Pin 13)"=w490:bool, "error out"=w495:errorcluster)
                  n179 = Not(x=w490) -> (.not. x?=w494:bool)
                  n180 = local write "Pin 13 State"(w490) -> ()
                  n181 = Or(x=w494, y=w489) -> (x .or. y?=w493:bool)
                }
                n182 = Or(x=w448, y=w447) -> (x .or. y?=→"LinkIt Response\nTimed Out 3":bool)
                n183 = xnode "Digital output (1 sample) 3"("A/DIO0 (Pin 11)"=w450, "error in (no error)"=w452) -> ("error out"=w451:errorcluster)
                n184 = local write "Pin 11 State"(w450) -> ()
              }
            }
          }
        }
        n185 = local read "Stop"() -> (w232:bool)
        n186 = Compound Arithmetic op=OR(w234, w235) -> (w233:bool)
        "M.S. Status" <- w233
        n187 = Or(x=w233, y=w232) -> (x .or. y?=w231:bool)
      }
      n188 = Release Queue(queue=w140, error in (no error)=w139) -> (error out=w131:errorcluster)  [unwired: 1 in, 2 out]
      n189 = Merge Errors(w130, w131) -> (w105:errorcluster)
      n190 = Release Queue(queue=w134, error in (no error)=w135) -> (error out=w127:errorcluster)  [unwired: 1 in, 2 out]
      n191 = Merge Errors(w123, w122, w121) -> (w109:errorcluster)
      n192 = Merge Errors(w114, w115, w120) -> (w107:errorcluster)
      n193 = Merge Errors(w127, w126) -> (w106:errorcluster)
      n194 = Release Queue(queue=w117, error in (no error)=w118) -> (error out=w112:errorcluster)  [unwired: 1 in, 2 out]
      n195 = Release Queue(queue=w133, error in (no error)=w132) -> (error out=w128:errorcluster)  [unwired: 1 in, 2 out]
      n196 = Merge Errors(w119, w112) -> (w108:errorcluster)
      n197 = Merge Errors(w128, w129) -> (w104:errorcluster)
      n198 = while {
        shift-right: [w830] -> _
        shift-left: w151 -> [w830]
        tunnel: [w811] -> w152
        stop <- w833 stop-if-true
        w815 = ":" ("string")
        w821 = 1
        # "method for calculating the uptime for the device measured in MM:DD:HH:MM:SS"
        # "System uptime"
        n199 = Get Date/Time In Seconds() -> (seconds since 1Jan1904=w834:timestamp)
        n200 = Wait (ms)(milliseconds to wait=u32 100) -> ()  [unwired: 1 out]
        n201 = Subtract(x=w834, y=w830) -> (x-y=w832:dbl)
        n202 = To Time Stamp(1:w832) -> (0:w814:timestamp)
        n203 = Get Date/Time String(seconds (now)=w814, want seconds? (F)=TRUE) -> (date string=w829:string)  [unwired: 1 in, 1 out]
        n204 = Match Pattern(string=w829, regular expression="/04") -> (before substring=w827:string)  [unwired: 1 in, 3 out]
        n205 = Match Pattern(string=w827, regular expression="/") -> (before substring=w825:string, after substring=w824:string)  [unwired: 1 in, 2 out]
        n206 = Decimal String To Number(string=w825) -> (number=w823:i32)  [unwired: 2 in, 1 out]
        n207 = Decimal String To Number(string=w824) -> (number=w822:i32)  [unwired: 2 in, 1 out]
        n208 = Subtract(x=w823, y=w821) -> (x-y=w819:i32)
        n209 = Subtract(x=w822, y=w821) -> (x-y=w820:i32)
        n210 = Number To Decimal String(number=w819) -> (decimal integer string=w818:string)  [unwired: 1 in]
        n211 = Number To Decimal String(number=w820) -> (decimal integer string=w817:string)  [unwired: 1 in]
        n212 = Format Date/Time String(time format string (%c)="%H:%M:%S", seconds (now)=w814) -> (date/time string=w812:string)  [unwired: 1 in]
        n213 = Concatenate Strings(w818, w815, w817, w815, w812) -> (w811:string)
        "System Uptime" <- w811
        n214 = local read "Stop"() -> (w833:bool)
      }
      n215 = Release Queue(queue=w137, error in (no error)=w136) -> (error out=w125:errorcluster)  [unwired: 1 in, 2 out]
      n216 = Merge Errors(w125, w124) -> (w103:errorcluster)
      n217 = Merge Errors(w110, w109, w108, w107, w106, w111, w105, w104, w103) -> (w101:errorcluster)
    }
    frame #2 {
      # "Close"
      n218 = call <vilib>:"Reset myRIO.vi"("error in (no error)"=w853) -> ("error out"=w856:errorcluster)  [unwired: 10 in]
      n219 = Unbundle By Name(w856) -> ("status"=w860:bool, "code"=w859:i32, "source"=w858:string)
      n220 = case shown="True" w860 {
        tunnel: w853 -> [w861 w883]
        tunnel: [w861 w881] -> w855
        tunnel: w859 -> [_ w870]
        tunnel: w858 -> [_ w867]
        tunnel: w854 -> [_ w864]
        tunnel: w857 -> [_ w863]
        frame False {
        }
        frame True {
          w868 = "\n"
          w874 = "\t"
          # "logs errors to the current log file"
          # "error logger"
          n221 = Number To Decimal String(number=w870) -> (decimal integer string=w871:string)  [unwired: 1 in]
          n222 = Number To Decimal String(number=0) -> (decimal integer string=w877:string)  [unwired: 1 in]
          n223 = Concatenate Strings("loop ", w877) -> (w875:string)
          n224 = Concatenate Strings("ERROR ", w871, "\r", w867) -> (w869:string)
          n225 = Open/Create/Replace File(file path (use dialog)=w864, error in=w883, operation (0:open)=T11."open or create") -> (refnum out=w886:refnum<file>, error out=w887:errorcluster)  [unwired: 3 in, 1 out]
          n226 = Format Date/Time String() -> (date/time string=w879:string)  [unwired: 3 in]
          n227 = Concatenate Strings(w879, w874, "\tLog Test" ("text"), w874, w875, w874, w868, w869, w868, "uptime" ("string"), w863) -> (w880:string)
          n228 = Set File Position(refnum=w886, from (0:start)=enum16{"start", "end", "current"}."end", error in=w887) -> (refnum out=w889:refnum<file>, error out=w888:errorcluster)  [unwired: 1 in]
          n229 = Write to Text File(file (use dialog)=w889, text=w880, error in=w888) -> (refnum out=w882:refnum<file>, error out=w865:errorcluster)  [unwired: 1 in, 1 out]
          n230 = Close File(refnum=w882, error in=w865) -> (error out=w881:errorcluster)  [unwired: 1 out]
        }
      }
      "error out" <- w855
    }
  }
